vi "Map Differential Pair.vi"(9 "Channel Pair Index":i32, 10 "Changed Channel Index":i32, 11 "Channel Definitions":cluster{"Channel":string, "Source":string}[](array[cluster])) -> (3 "Channel Definitions":cluster{"Channel":string, "Source":string}[](array[cluster]))   [LabVIEW 2020, in "Routing and Faulting System Explorer.lvlib"]
uses:
  Routing and Faulting System Explorer.lvlib
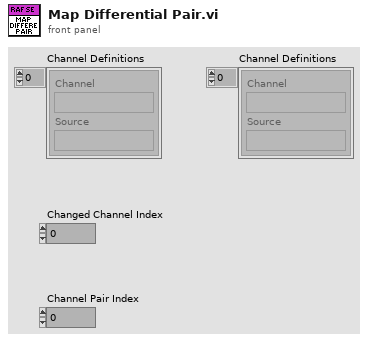
[diagram p1: front panel]
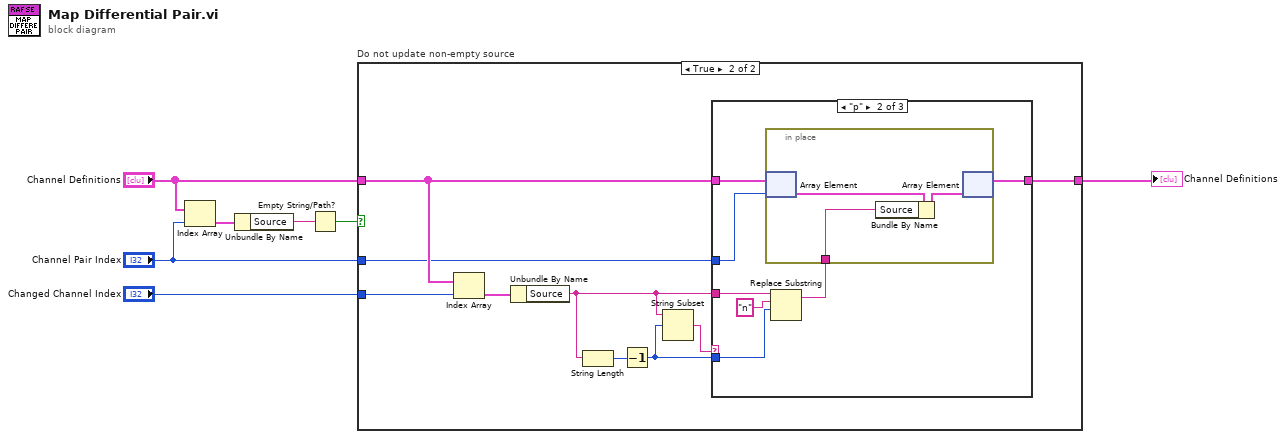
[diagram p0: block diagram]
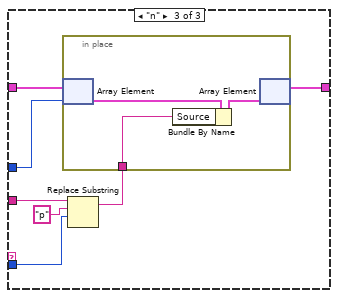
[diagram p4: hidden frame]
diagram:
  n1 = Index Array(array="Channel Definitions", index="Channel Pair Index") -> (element=w3:cluster{"Channel":string, "Source":string})
  n2 = Unbundle By Name(w3) -> ("Source"=w2:string)
  n3 = Empty String/Path?(string/path=w2) -> (empty?=w1:bool)
  n4 = case "Do not update non-empty source" shown="True" w1 {
    tunnel: "Changed Channel Index" -> [_ w17]
    tunnel: "Channel Definitions" -> [w8 w13]
    tunnel: [w8 w12] -> w6
    tunnel: "Channel Pair Index" -> [_ w10]
    frame False {
    }
    frame True {
      n5 = Index Array(array=w13, index=w17) -> (element=w16:cluster{"Channel":string, "Source":string})
      n6 = Unbundle By Name(w16) -> ("Source"=w11:string)
      n7 = String Length(string=w11) -> (length=w15:i32)
      n8 = Decrement(x=w15) -> (x-1=w9:i32)
      n9 = String Subset(string=w11, offset (0)=w9) -> (substring=w14:string)  [unwired: 1 in]
      n10 = case shown="\"p\"" w14 {
        tunnel: w13 -> [w18 w25 w35]
        tunnel: [w18 w20 w30] -> w12
        tunnel: w11 -> [_ w23 w33]
        tunnel: w10 -> [_ w24 w34]
        tunnel: w9 -> [_ w22 w32]
        frame "", Default {
        }
        frame "p" {
          n11 = Replace Substring(3:w22, 4:"n" ("substring (\"\")"), 5:w23) -> (1:w19:string)  [unwired: 1 in, 1 out]
          n12 = in-place {
            in-place-border: w19 -> [w26]
            n13 = in-place-array #1(w25, w24) -> (w28:cluster{"Channel":string, "Source":string})
            n14 = Bundle By Name(cluster=w28, "Source"=w26) -> (w27:cluster{"Channel":string, "Source":string})
            n15 = in-place-array #1(w27) -> (w20:cluster{"Channel":string, "Source":string}[])  [unwired: 1 out]
          }
        }
        frame "n" {
          n16 = Replace Substring(3:w32, 4:"p" ("substring (\"\")"), 5:w33) -> (1:w29:string)  [unwired: 1 in, 1 out]
          n17 = in-place {
            in-place-border: w29 -> [w36]
            n18 = in-place-array #2(w35, w34) -> (w38:cluster{"Channel":string, "Source":string})
            n19 = Bundle By Name(cluster=w38, "Source"=w36) -> (w37:cluster{"Channel":string, "Source":string})
            n20 = in-place-array #2(w37) -> (w30:cluster{"Channel":string, "Source":string}[])  [unwired: 1 out]
          }
        }
      }
    }
  }
  "Channel Definitions" <- w6
